vi "QuerySystemSession.vi"(8 "error in (no error)":errorcluster) -> (0 "error out":errorcluster)   [LabVIEW 2017, in "SystemInfoProcess.lvlib"]
uses:
  <vilib>/addons/SystemInfoProcess/SystemInfoProcess.lvlib
  <vilib>/nisyscfg/nisyscfg.lvlib
  <vilib>/nisyscfg/Close (System).vi
  <resource>/objmgr/nisysapi.rc
  <vilib>/addons/PointValueMap/PointValueMap.lvlib
  <vilib>/addons/PointValueMap/subVIs/Point_Write_string.vi
  <vilib>/addons/PointValueMap/subVIs/Point_Write_variant.vi
  <vilib>/addons/SystemInfoProcess/controls/ImageMetadata.ctl
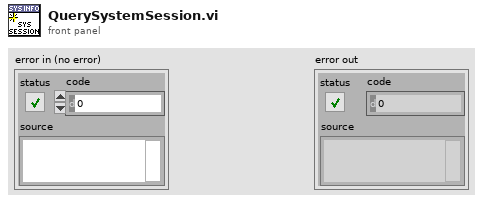
[diagram p1: front panel]
types:
  T1 = typedef "SystemInfoProcess.lvlib/ImageMetadata.ctl" = cluster{"Title":string, "Description":string, "ID":string, "Version":string}
  T2 = typedef "PointValueMap.lvlib/PointMap.ctl" = refnum<data-value>
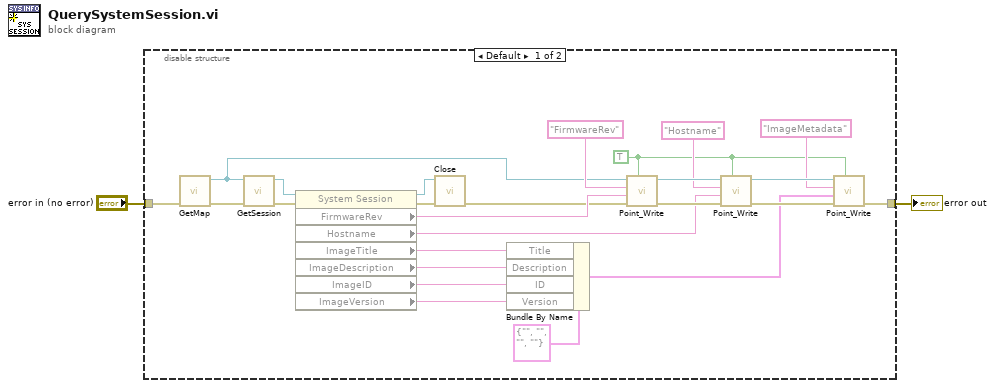
[diagram p0: block diagram]
diagram:
  n1 = disable-structure shown="Default" {
    disable-tunnel: "error in (no error)" -> [w7 w28]
    disable-tunnel: [w18 w28] -> w1
    frame condition #0 {
      w19 = TRUE ("Auto Create?")
      n2 = call <vilib>:"GetMap.vi"("error in (no error)"=w7) -> ("error out"=w8:errorcluster, "SystemInfoMap"=w4:T2)  [unwired: 9 in]
      n3 = call <vilib>:"GetSession.vi"("error in (no error)"=w8, "map"=w4) -> ("error out"=w6:errorcluster, "session"=w5:refnum<k21>)  [unwired: 8 in]
      n4 = property class="System Session"(reference=w5, error in=w6) -> (reference out=w27:refnum<k21>, error out=w26:errorcluster, "FirmwareRev"=w16:string, "Hostname"=w15:string, "ImageTitle"=w13:string, "ImageDescription"=w12:string, "ImageID"=w11:string, "ImageVersion"=w10:string)
      n5 = call-poly <vilib>:"Close.vi"("error in (no error)"=w26, "Session in"=w27) -> ("error out"=w3:errorcluster)  [unwired: 9 in]
      n6 = Bundle By Name(cluster=T1 {"Title"="", "Description"="", "ID"="", "Version"=""} ("ImageMetadata"), "Title"=w13, "Description"=w12, "ID"=w11, "Version"=w10) -> (w9:T1)
      n7 = call-poly <vilib>:"Point_Write.vi"("Auto Create?"=w19, "Error In"=w3, "Value"=w16, "Tag"="FirmwareRev", "Map"=w4) -> ("Error Out"=w25:errorcluster, "Map Out"=w24:T2)  [unwired: 5 in]
      n8 = call-poly <vilib>:"Point_Write.vi"("Auto Create?"=w19, "Error In"=w25, "Value"=w15, "Tag"="Hostname", "Map"=w24) -> ("Error Out"=w22:errorcluster, "Map Out"=w21:T2)  [unwired: 5 in]
      n9 = call-poly <vilib>:"Point_Write.vi"("Auto Create?"=w19, "Error In"=w22, "Value"=w9, "Tag"="ImageMetadata", "Map"=w21) -> ("Error Out"=w18:errorcluster)  [unwired: 5 in, 1 out]
    }
    frame condition #1 (active) {
    }
  }
  "error out" <- w1
